vi "Initialize Hardware References.vi"(8 "error in":errorcluster, 11 "HW Refnum in":string) -> (0 "error out":errorcluster, 3 "HW Refnum out":string)   [LabVIEW 2025, in "Acquisition.lvlib"]
doc: "Initialize the hardware references.\n_____\nBased on DQMH Dev Tools: Project Template 7.1.0.1503."
uses:
  Acquisition.lvlib
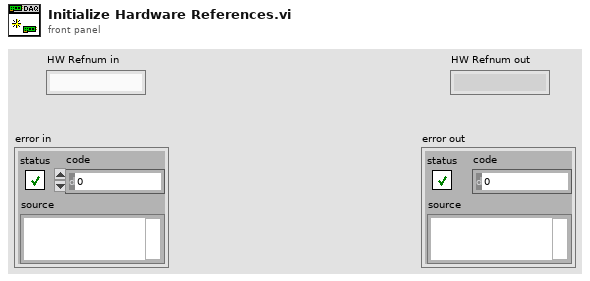
[diagram p1: front panel]
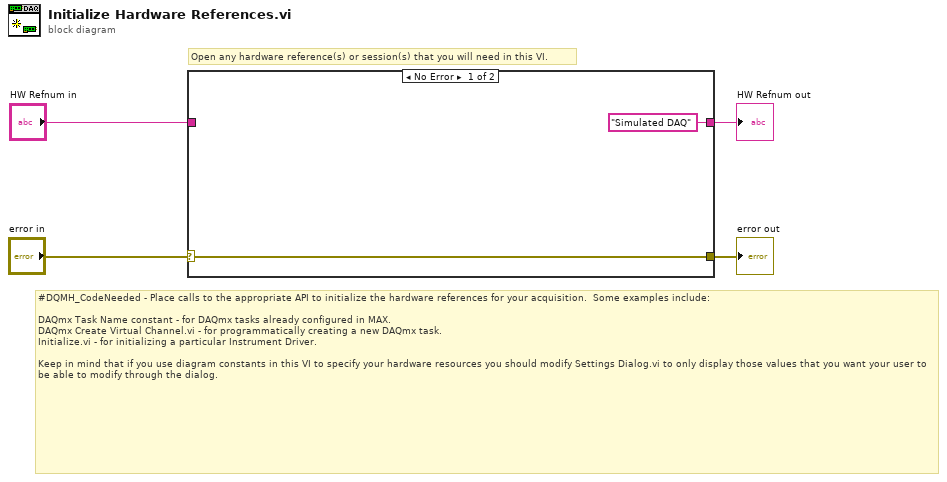
[diagram p0: block diagram]
diagram:
  # "Open any hardware reference(s) or session(s) that you will need in this VI."
  # "#DQMH_CodeNeeded - Place calls to the appropriate API to initialize the hardware references for your acquisition.  Some examples include:\n\nDAQmx Task Name constant - for DAQmx tasks already configured in MAX.\nDAQmx Create Virtual Channel.vi - for programmatically creating a new DAQmx task.\nInitialize.vi - for initializing a particular Instrument Driver.\n\nKeep in mind that if you use diagram constants in this VI to specify your hardware resources you should modify Settings Dialog.vi to only display those values that you want your user to be able to modify through the dialog."
  n1 = case shown="No Error" "error in" {
    selector: "error in" -> [w6 w7]
    tunnel: [w6 w7] -> w3
    tunnel: "HW Refnum in" -> [_ w8]
    tunnel: ["Simulated DAQ" ("HW Refnum in") w8] -> w1
    frame No Error {
    }
    frame Error {
    }
  }
  "HW Refnum out" <- w1
  "error out" <- w3
